vi "Read FunctionClass.vi"(8 "error in (no error)":errorcluster, 11 "FgenPluginsBase in":refnum<class "FgenPluginsBase.lvclass">) -> (0 "error out":errorcluster, 2 "Functions.lvlib:FunctionBase.lvclass":refnum<class "FunctionBase.lvclass">, 3 "FgenPluginsBase out":refnum<class "FgenPluginsBase.lvclass">)   [LabVIEW 2014, in "FgenPlugins.lvlib" / "FgenPluginsBase.lvclass"]
uses:
  FgenPluginsBase.lvclass
  MemberClasses/FunctionBaseClass/FunctionBase.lvclass
  FgenPluginsBase.lvclass/FgenPluginsBase.ctl
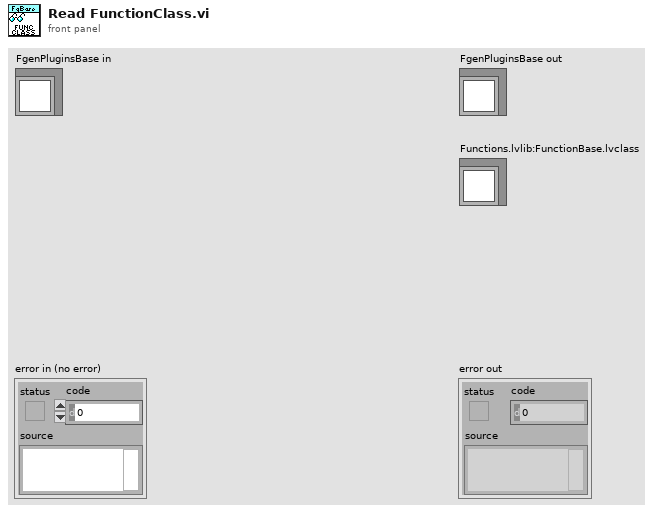
[diagram p1: front panel]
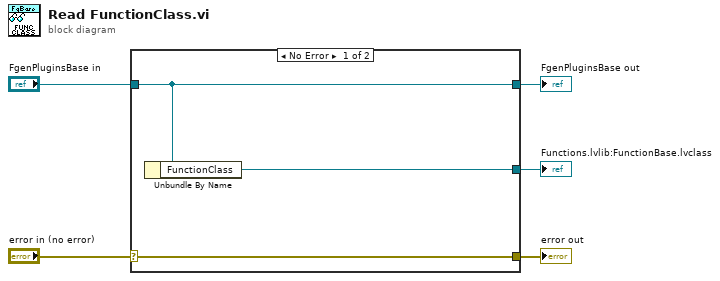
[diagram p0: block diagram]
diagram:
  n1 = case shown="No Error" "error in (no error)" {
    selector: "error in (no error)" -> [w8 w9]
    tunnel: [w8 w9] -> w4
    tunnel: [w7 w10] -> w2
    tunnel: "FgenPluginsBase in" -> [w7 w10]
    tunnel: [w6 _] -> w1
    frame No Error {
      n2 = Unbundle By Name(w7) -> ("FunctionClass"=w6:refnum<class "FunctionBase.lvclass">)
    }
    frame Error {
    }
  }
  "error out" <- w4
  "FgenPluginsBase out" <- w2
  "Functions.lvlib:FunctionBase.lvclass" <- w1
